vi "Image Global Counter.vi"() -> ()   [LabVIEW 2015]
panel:
  in  "Image Counter":u64
  # "As Image read from Camera This counter keeps Increamenting\nIndividual Counter is there per Camera"
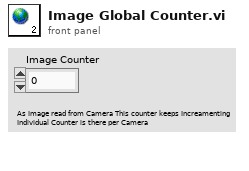
[diagram p1: front panel]
diagram:
